vi "overstack.vi"(9 "board array":i16[][](array[numeric]), 11 "Piece Array":i16[][](array[numeric])) -> (1 "min Distance":i16, 2 "Lost":bool, 3 "Touching":bool)   [LabVIEW 2018]
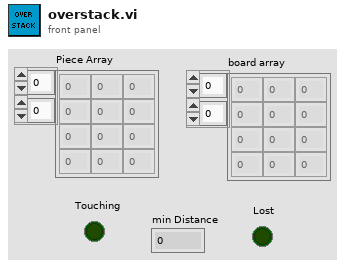
[diagram p1: front panel]
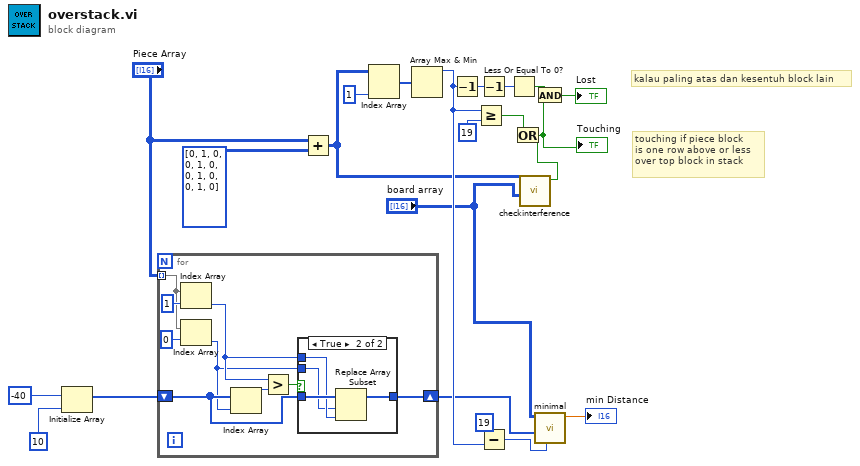
[diagram p0: block diagram]
diagram:
  # "touching if piece block\nis one row above or less \nover top block in stack"
  # "kalau paling atas dan kesentuh block lain"
  n1 = Initialize Array(i16 -40, 10) -> (w20:i16[])
  n2 = for {
    tunnel: "Piece Array" -> [w29] mode=indexing
    shift-right: [w26] -> w6
    shift-left: w20 -> [w25]
    n3 = Index Array(array=w29, index=1) -> (element=w24:i16)
    n4 = Index Array(array=w29, index=0) -> (element=w23:i16)
    n5 = Index Array(array=w25, index=w23) -> (element=w28:i16)
    n6 = Greater?(x=w24, y=w28) -> (0:w27:bool)
    n7 = case shown="True" w27 {
      tunnel: [w32 w36] -> w26
      tunnel: w25 -> [w32 w35]
      tunnel: w24 -> [_ w34]
      tunnel: w23 -> [_ w33]
      frame False {
      }
      frame True {
        n8 = Replace Array Subset(array=w35, new element=w34, index=w33) -> (w36:i16[])
      }
    }
  }
  n9 = Add(x="Piece Array", y=i32[][] [[0, 1, 0], [0, 1, 0], [0, 1, 0], [0, 1, 0]]) -> (x+y=w3:i32[][])
  n10 = Index Array(array=w3, index (col)=1) -> (element=w16:i32[])  [unwired: 1 in]
  n11 = Array Max & Min(array=w16) -> (max value=w8:i32)  [unwired: 3 out]
  n12 = Decrement(x=w8) -> (x-1=w15:i32)
  n13 = Greater Or Equal?(x=w8, y=19) -> (x >= y?=w10:bool)
  n14 = Decrement(x=w15) -> (x-1=w7:i32)
  n15 = Subtract(x=19, y=w8) -> (x-y=w5:i32)
  n16 = Less Or Equal To 0?(x=w7) -> (x <= 0?=w14:bool)
  n17 = call "checkinterference.vi"(9:"board array", "piece"=w3) -> (3:w1:bool)  [unwired: 9 in]
  n18 = Or(x=w10, y=w1) -> (x .or. y?=w9:bool)
  "Touching" <- w9
  n19 = And(x=w14, y=w9) -> (x .and. y?=→"Lost":bool)
  n20 = call "minimal.vi"("Numeric"=w5, "Array"=w6, "Array 2"="board array") -> ("Numeric 2"=→"min Distance":dbl)  [unwired: 8 in]
